vi "Render Recursive Partial with Multiple Recursion.vi"(8 "Error In":errorcluster) -> (0 "Error Out":errorcluster)   [LabVIEW 2018, in "Tests.lvlib" / "Render.lvlib"]
uses:
  Render.lvlib
  src/Toolkit/Data/Map/Map.lvclass
  D:/Users/cfield/Code/Field R&D Services/Labstache/src/Toolkit/Data/Datum/Datum.lvclass
  src/Toolkit/Data/Array/Array.lvclass
  src/Toolkit/Low-Level/Loaders/String/String.lvclass
  D:/Users/cfield/Code/Field R&D Services/Labstache/src/Toolkit/Low-Level/Loaders/Loader/Loader.lvclass
  src/Toolkit/Low-Level/Support/Lex String.vi
  src/Toolkit/Data/Pair/Support/From String.vi
  src/Toolkit/Data/Pair/Support/From Boolean.vi
  src/Toolkit/Data/Map/Support/From Pair Array.vi
  src/Toolkit/Data/Array/Support/From Data.vi
  src/Toolkit/Data/Pair/Support/From Datum.vi
  src/Toolkit/Low-Level/Support/Render to String.vi
  <vilib>/addons/_JKI Toolkits/Caraya/classes/Test/Test.lvclass
  <vilib>/addons/_JKI Toolkits/Caraya/classes/Assert/Assert.lvclass
  src/Toolkit/Toolkit.lvlib
  src/Toolkit/Data/Pair/Pair.lvclass
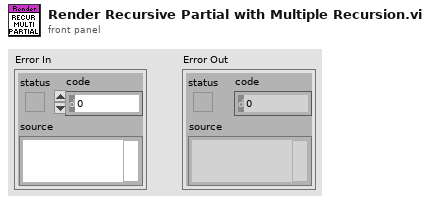
[diagram p1: front panel]
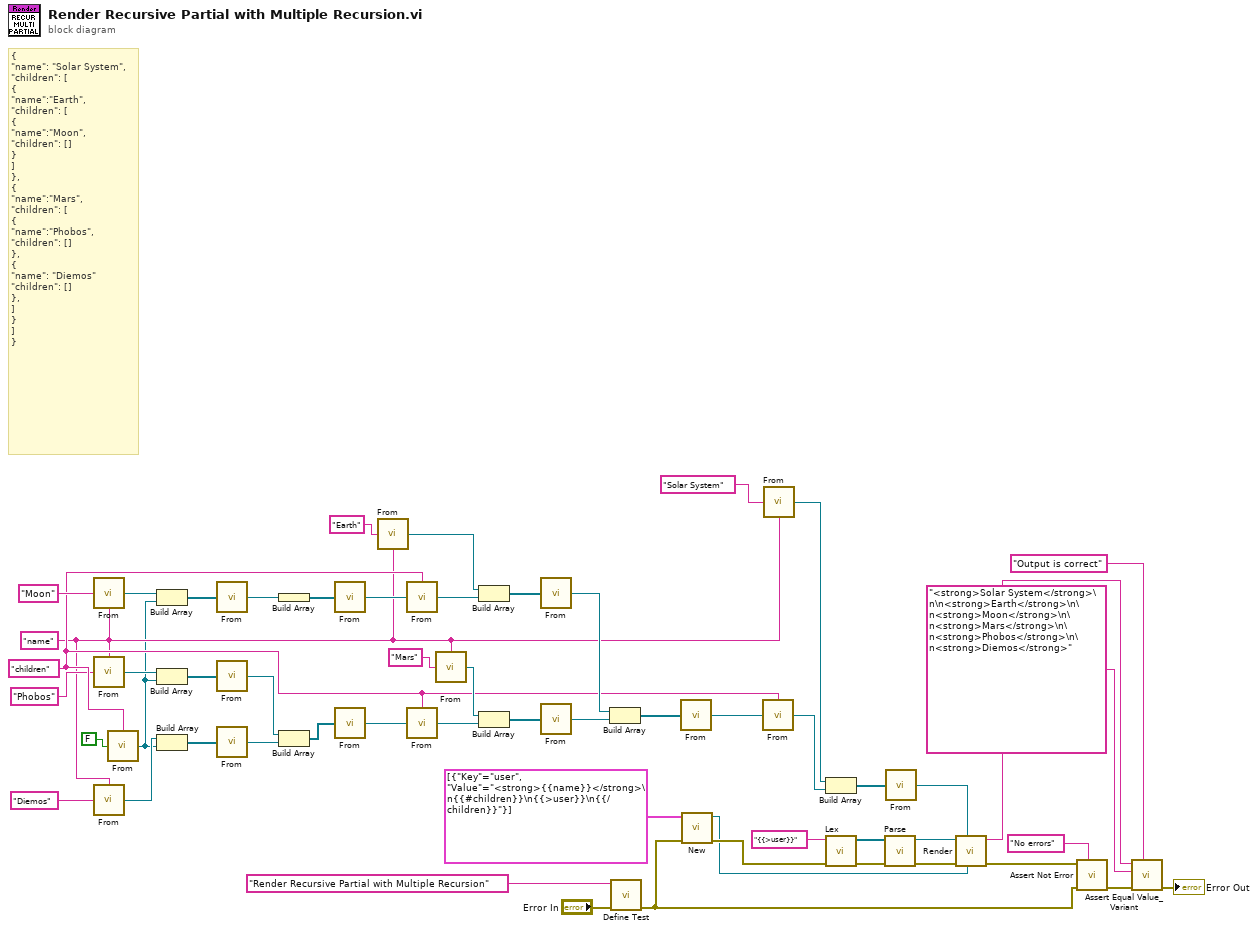
[diagram p0: block diagram]
diagram:
  w18 = "children" ("Key")
  w5 = "name" ("Key")
  # "{\n\"name\": \"Solar System\",\n\"children\": [\n{\n\"name\":\"Earth\",\n\"children\": [\n{\n\"name\":\"Moon\",\n\"children\": []\n}\n]\n},\n{\n\"name\":\"Mars\",\n\"children\": [\n{\n\"name\":\"Phobos\",\n\"children\": []\n},\n{\n\"name\": \"Diemos\"\n\"children\": []\n},\n]\n}\n]\n}"
  n1 = call-poly "From.vi"("Value"="Moon", "Key"=w5) -> ("Pair"=w16:refnum<class "Pair.lvclass">)
  n2 = call-poly "From.vi"("Value"="Phobos", "Key"=w5) -> ("Pair"=w3:refnum<class "Pair.lvclass">)
  n3 = call-poly "From.vi"("Value"="Diemos", "Key"=w5) -> ("Pair"=w2:refnum<class "Pair.lvclass">)
  n4 = call-poly "From.vi"("Value"=FALSE, "Key"=w18) -> ("Pair"=w1:refnum<class "Pair.lvclass">)
  n5 = Build Array(w16, w1) -> (w15:refnum<class "Pair.lvclass">[])
  n6 = Build Array(w3, w1) -> (w8:refnum<class "Pair.lvclass">[])
  n7 = Build Array(w2, w1) -> (w7:refnum<class "Pair.lvclass">[])
  n8 = call-poly "From.vi"("Pairs"=w15) -> ("Map"=w14:refnum<class "Map.lvclass">)  [unwired: 1 in]
  n9 = call-poly "From.vi"("Pairs"=w8) -> ("Map"=w10:refnum<class "Map.lvclass">)  [unwired: 1 in]
  n10 = call-poly "From.vi"("Pairs"=w7) -> ("Map"=w9:refnum<class "Map.lvclass">)  [unwired: 1 in]
  n11 = Build Array(w14) -> (w13:refnum<class "Map.lvclass">[])
  n12 = Build Array(w10, w9) -> (w11:refnum<class "Map.lvclass">[])
  n13 = call-poly "From.vi"("Data"=w13) -> ("Array"=w12:refnum<class "Array.lvclass">)  [unwired: 1 in]
  n14 = call-poly "From.vi"("Data"=w11) -> ("Array"=w20:refnum<class "Array.lvclass">)  [unwired: 1 in]
  n15 = call-poly "From.vi"("Value"="Earth", "Key"=w5) -> ("Pair"=w29:refnum<class "Pair.lvclass">)
  n16 = call-poly "From.vi"("Value"=w12, "Key"=w18) -> ("Pair"=w28:refnum<class "Pair.lvclass">)
  n17 = call-poly "From.vi"("Value"=w20, "Key"=w18) -> ("Pair"=w23:refnum<class "Pair.lvclass">)
  n18 = call-poly "From.vi"("Value"="Mars", "Key"=w5) -> ("Pair"=w24:refnum<class "Pair.lvclass">)
  n19 = Build Array(w29, w28) -> (w27:refnum<class "Pair.lvclass">[])
  n20 = Build Array(w24, w23) -> (w22:refnum<class "Pair.lvclass">[])
  n21 = call-poly "From.vi"("Pairs"=w27) -> ("Map"=w26:refnum<class "Map.lvclass">)  [unwired: 1 in]
  n22 = call-poly "From.vi"("Pairs"=w22) -> ("Map"=w21:refnum<class "Map.lvclass">)  [unwired: 1 in]
  n23 = Build Array(w26, w21) -> (w35:refnum<class "Map.lvclass">[])
  n24 = call <vilib>:"Define Test.vi"("error in (no error)"="Error In", "Label (VI Title)"="Render Recursive Partial with Multiple Recursion") -> ("error out"=w41:errorcluster)  [unwired: 9 in]
  n25 = call-poly "From.vi"("Data"=w35) -> ("Array"=w34:refnum<class "Array.lvclass">)  [unwired: 1 in]
  n26 = call "New.vi"("Error In"=w41, "Key-Value Pairs"=cluster{"Key":string, "Value":string}[] [{"Key"="user", "Value"="<strong>{{name}}</strong>\n{{#children}}\n{{>user}}\n{{/children}}"}]) -> ("Error Out"=w43:errorcluster, "String"=w38:refnum<class "String.lvclass">)  [unwired: 8 in]
  n27 = call-poly "From.vi"("Value"=w34, "Key"=w18) -> ("Pair"=w32:refnum<class "Pair.lvclass">)
  n28 = call-poly "From.vi"("Value"="Solar System", "Key"=w5) -> ("Pair"=w33:refnum<class "Pair.lvclass">)
  n29 = Build Array(w33, w32) -> (w31:refnum<class "Pair.lvclass">[])
  n30 = call-poly "Lex.vi"("Error In"=w43, "Input"="{{>user}}" ("format string")) -> ("Error Out"=w45:errorcluster, "Tokens"=w46:refnum<class "Token.lvclass">[])  [unwired: 8 in]
  n31 = call "Parse.vi"("Error In"=w45, "Tokens"=w46) -> ("Error Out"=w47:errorcluster, "Abstract Syntax Tree"=w44:refnum<class "Root.lvclass">)  [unwired: 8 in]
  n32 = call-poly "From.vi"("Pairs"=w31) -> ("Map"=w30:refnum<class "Map.lvclass">)  [unwired: 1 in]
  n33 = call-poly "Render.vi"("Loader"=w38, "Data"=w30, "Error In"=w47, "Abstract Syntax Tree"=w44) -> ("Error Out"=w49:errorcluster, "Output"=w48:string)  [unwired: 6 in]
  n34 = call <vilib>:"Assert Not Error.vi"("Label"="No errors", "error in (no error)"=w41, "Not Error?"=w49) -> ("error out"=w52:errorcluster)  [unwired: 8 in]
  n35 = call <vilib>:"Assert Equal Value_Variant.vi"("Label"="Output is correct", "error in (no error)"=w52, "Y"="<strong>Solar System</strong>\n\n<strong>Earth</strong>\n\n<strong>Moon</strong>\n\n<strong>Mars</strong>\n\n<strong>Phobos</strong>\n\n<strong>Diemos</strong>", "X"=w48) -> ("error out"=→"Error Out":errorcluster)  [unwired: 7 in]
